vi "Remove Unconfigured DAQmx Devices.vi"(8 "error in (no error)":errorcluster) -> (0 "error out":errorcluster)   [LabVIEW 2011]
uses:
  DLLs/autoconf.dll
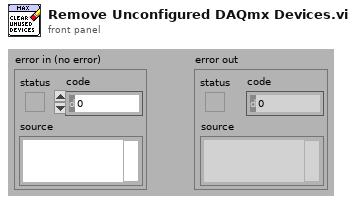
[diagram p1: front panel]
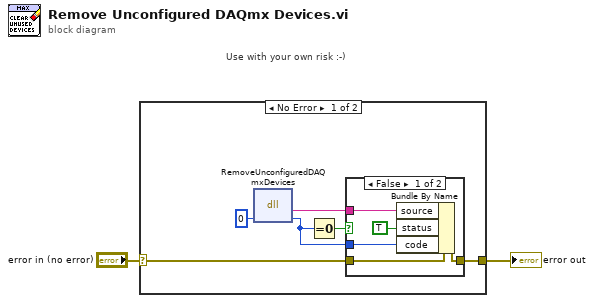
[diagram p0: block diagram]
diagram:
  # "Use with your own risk :-)"
  n1 = case shown="No Error" "error in (no error)" {
    selector: "error in (no error)" -> [w7 w15]
    tunnel: [w6 w15] -> w2
    frame No Error {
      n2 = dll-call lib="C:/Users/fibergss/Desktop/cDAQ Finder/DLLs/autoconf.dll" fn="RemoveUnconfiguredDAQmxDevices"("Status"=0) -> ("return type"=w4:string, "Status"=w3:i32)  [unwired: 3 in, 2 out]
      n3 = Equal To 0?(x=w3) -> (x = 0?=w8:bool)
      n4 = case shown="False" w8 {
        tunnel: w7 -> [w13 w14]
        tunnel: [w12 w14] -> w6
        tunnel: w4 -> [w10 _]
        tunnel: w3 -> [w9 _]
        frame False {
          n5 = Bundle By Name(cluster=w13, "source"=w10, "status"=TRUE, "code"=w9) -> (w12:errorcluster)
        }
        frame True {
        }
      }
    }
    frame Error {
    }
  }
  "error out" <- w2
